vi "Fire UpdateControlValue Event.vi"(8 "error in (no error)":errorcluster, 9 "vData":variant, 10 "Control Label":string, 11 "Main in":refnum<class "Main.lvclass">) -> (0 "error out":errorcluster, 3 "Main out":refnum<class "Main.lvclass">)   [LabVIEW 2019, in "Main.lvclass"]
doc: "Developed by Kevin Thompson\nkevin@thompsonengineering.net\n\nCopyright 2018\nThompson Engineering, LLC"
uses:
  Main.lvclass
  Common/DataTypes/UpdateControlValue EvData--cluster.ctl
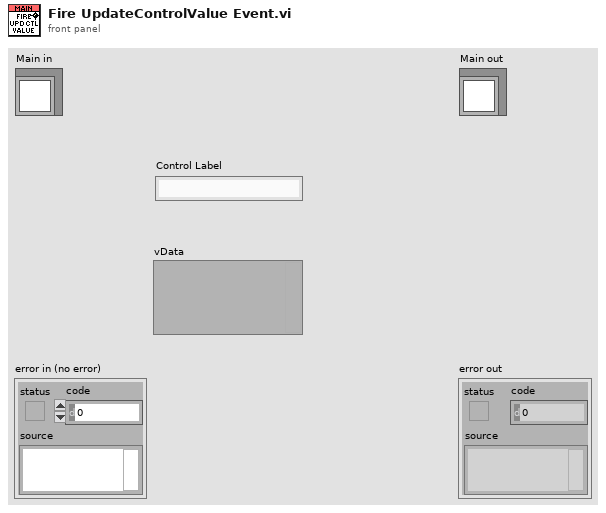
[diagram p1: front panel]
types:
  T1 = typedef "UpdateControlValue EvData--cluster.ctl" = cluster{"Time Stamp":timestamp, "ControlLabel":string, "vData":variant}
  T2 = typedef "Main.lvclass/Public Events--cluster.ctl" = cluster{"Main.AsyncCmd Event":refnum<user-event>, "Main.AsyncMsg Event":refnum<user-event>, "stop process":refnum<user-event>, "UpdateControlValue Ev":refnum<user-event>, "ProcessingStateChg Ev":refnum<user-event>}
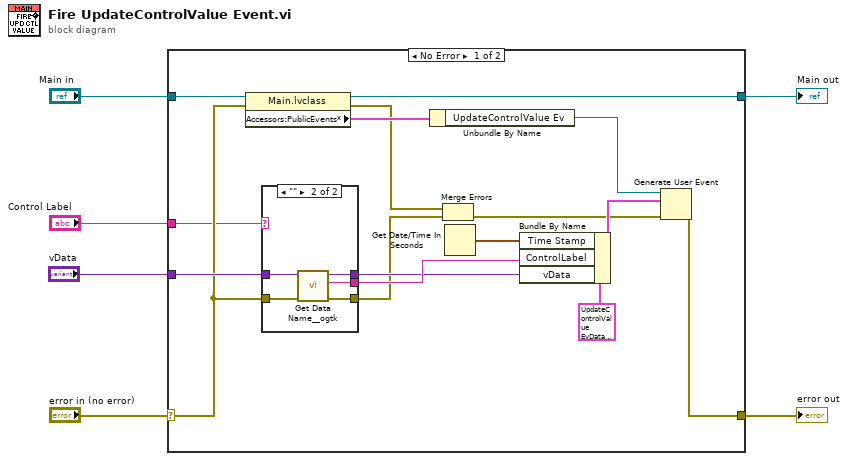
[diagram p0: block diagram]
diagram:
  n1 = case shown="No Error" "error in (no error)" {
    selector: "error in (no error)" -> [w8 w32]
    tunnel: [w22 w32] -> w5
    tunnel: [w17 w31] -> w3
    tunnel: "Main in" -> [w18 w31]
    tunnel: "vData" -> [w11 _]
    tunnel: "Control Label" -> [w7 _]
    frame No Error {
      n2 = property class="Main.lvclass"(reference=w18, error in=w8) -> (reference out=w17:refnum<class "Main.lvclass">, error out=w14:errorcluster, "Accessors:PublicEvents*"=w19:T2)
      n3 = case shown="\"\"" w7 {
        selector: w7 -> [w25 _]
        tunnel: [w25 w30] -> w13
        tunnel: [w24 w29] -> w12
        tunnel: w11 -> [w24 w28]
        tunnel: [w23 w27] -> w9
        tunnel: w8 -> [w23 w26]
        frame Default {
        }
        frame "" {
          n4 = call <userlib>:"Get Data Name__ogtk.vi"("error in (no error)"=w26, "Data"=w28) -> ("error out"=w27:errorcluster, "Data Name"=w30:string, "Data dup"=w29:variant)  [unwired: 7 in]
        }
      }
      n5 = Unbundle By Name(w19) -> ("UpdateControlValue Ev"=w16:refnum<user-event>)
      n6 = Merge Errors(w14, w9) -> (w15:errorcluster)
      n7 = Get Date/Time In Seconds() -> (seconds since 1Jan1904=w20:timestamp)
      n8 = Bundle By Name(cluster=T1 {"Time Stamp"=timestamp(0 s since 1904-01-01), "ControlLabel"="", "vData"=variant} ("UpateControlValue EvData"), "Time Stamp"=w20, "ControlLabel"=w13, "vData"=w12) -> (w21:T1)
      n9 = Generate User Event(user event=w16, event data cluster=w21, error in=w15) -> (error out=w22:errorcluster)  [unwired: 1 in, 1 out]
    }
    frame Error {
    }
  }
  "error out" <- w5
  "Main out" <- w3
